vi "Set Sheet Name.vi"(6 "Sheet Name (Sheet1)":string="Sheet1", 7 "Sheet":i32, 8 "error in (no error)":errorcluster, 11 "Workbook Reference":refnum<k24>) -> (0 "error out":errorcluster, 3 "Workbook Reference":refnum<k24>)   [LabVIEW 2013]
uses:
  C:/PhaeronGit/LVNPOI/Resources/NPOI 2.1.1 dotnet2/NPOI.dll
  Resources/NPOI 2.1.1 dotnet2/NPOI.dll
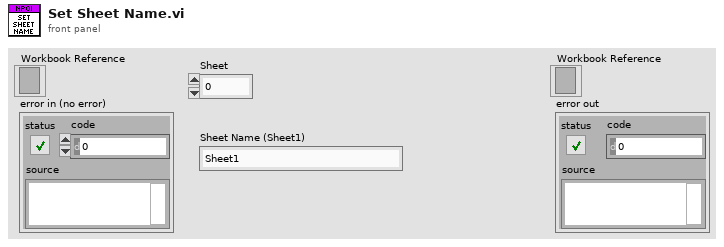
[diagram p1: front panel]
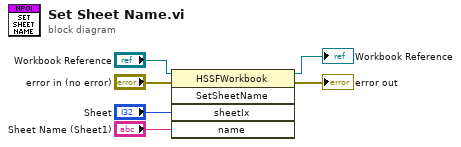
[diagram p0: block diagram]
diagram:
  n1 = invoke class="HSSFWorkbook" method="SetSheetName"(reference="Workbook Reference", error in="error in (no error)", "sheetIx"="Sheet", "name"="Sheet Name (Sheet1)") -> (reference out=→"Workbook Reference":refnum<k24>, error out=→"error out":errorcluster)  [unwired: 1 in, 3 out]
